vi "lm Get LE State.vi"(8 "error in (no error)":errorcluster) -> (0 "error out":errorcluster, 3 "function return":i32)   [LabVIEW 2017, in "LumencorDLLDbg64.lvlib"]
doc: "The Get LE State function is used with Sola and SolaSE light engines only. This call will return the LE Color Level and Enable state. The value returned will be an integer that contains both the enable state and Level info. \nSee DLL documentation for more detail.\n\n\nextern \"C\" LUMENCORDLL2B_API int lmGetLEState(void);"
uses:
  LumencorDLLDbg64.lvlib
  LumencorDLLDbg64.dll
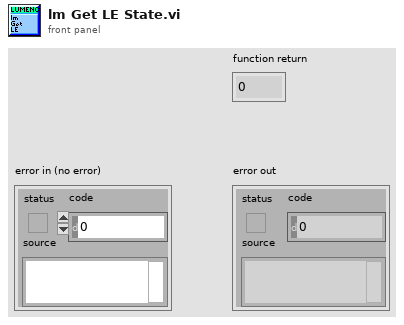
[diagram p1: front panel]
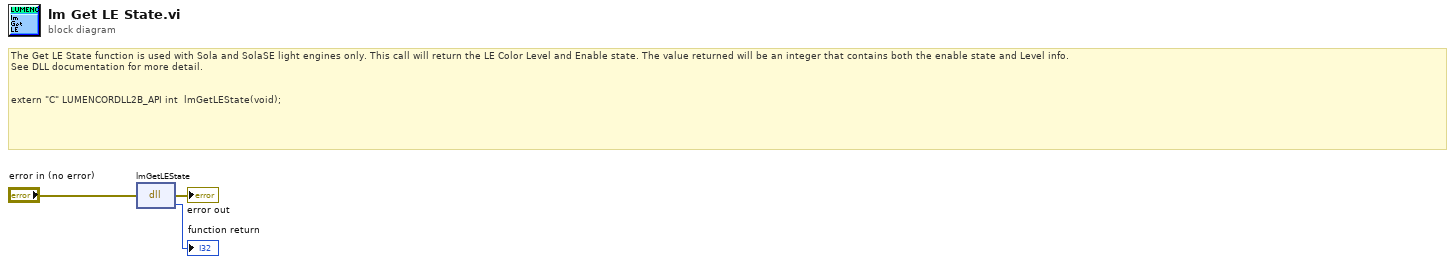
[diagram p0: block diagram]
diagram:
  # "The Get LE State function is used with Sola and SolaSE light engines only. This call will return the LE Color Level and Enable state. The value returned will be an integer that contains both the enable state and Level info. \nSee DLL documentation for more detail.\n\n\nextern \"C\" LUMENCORDLL2B_API int  lmGetLEState(void);"
  n1 = dll-call lib="Q:/GIT -- Lumencor DLL4/LabVIEW Library (64bit)/LumencorDLLDbg64.*" fn="lmGetLEState"(error in="error in (no error)") -> (error out=→"error out":errorcluster, →"function return":i32)  [unwired: 2 in, 1 out]
